vi "Chart_Generation_Formula.vi"(3 "Max Voltage":dbl, 7 "error in (no error)":errorcluster, 8 "Start":bool, 9 "CGF_Input":refnum<vi>, 10 "Polarity for Max Voltage":u16(ring) items=["Positive", "Negative"], 11 "Type of Chart":u16(ring) items=[" Crude Semi-Log (Short)", "Crude Semi-Log (Long)", "Bi-directional Crude Semi-Log (Short)", "Bi-directional Crude Semi-Log (Long)"]) -> (0 "Result - Test Voltages Array":dbl[](array[numeric]), 1 "~~ FINISH ~~":bool, 5 "error out":errorcluster)   [LabVIEW 2020]
uses:
  Global 1.vi
panel:
  out "Array Size":i32
  out "BiD : Test Voltages <OUTPUT>":dbl[](array[numeric])
  out "first subarray : PosTestV":dbl[](array[numeric])
  out "reversed array : NegTestV":dbl[](array[numeric])
  out "Flag Formula LCLC":bool
  out "Flag Formula SCLC":bool
  out "Checking NumberOfVoltages":i32
  out "DONE SUB Bi-LCLC":bool
  in  "SUB Bi-LCLC":bool
  out "DONE SUB Bi-SCLC":bool
  in  "SUB Bi-SCLC":bool
  out "BIDIRECTIONAL = FINISH Formulating Test Voltages":bool
  out "Bi-directional Crude Semi-Log (Long)":bool
  out "Bi-directional Crude Semi-Log (Short)":bool
  out "Crude Semi-Log (Long)":bool
  out "Crude Semi-Log (Short)":bool
  out "NegativeVoltages[256]":dbl[](array[numeric])
  out "Negative value":dbl
  in  "NumberOfVoltages":i32
  out "DONE SUB LCLC":bool
  in  "SUB LCLC":bool
  out "UNIDIRECTIONAL - FINISH Formulating Test Voltages":bool
  out "DONE SUB SCLC":bool
  in  "SUB SCLC":bool
  out "UniD : Test Voltages <OUTPUT>":dbl[](array[numeric])
  out "Checking Value of X":i32
  out "PositiveVoltages[256]":dbl[](array[numeric])
  in  "x":i32
  in  "VRmax":dbl
  # "Type of Chart :\n\n1) Linear -  < not applied here > < directly in Generation Report VI >\n2) Crude Semi-Log (Short) -----------------------> 0 \n3) Crude Semi-Log (Long) -----------------------> 1\n4) Bi-directional Crude Semi-Log (Short) --------> 2\n5) Bi-directional Crude Semi-Log (Long) --------> 3"
  # "FOR"
  # "Bi-directional Crude Semi-Log (Short)"
  # "Bi-directional Crude Semi-Log (Long)"
  # "Polarity is applied for \nmaximum voltage only,\nno mention of minimum\nin QuickBasic Code"
  # "Polarity : \n1 = \"negative\" ; 0 = \"positive\""
  # "Max Voltage is the actual\nmaximum voltage from\ndatasheet, therefore,\nmust put (-) if negative"
  # "VRmax is for calculation purpose"
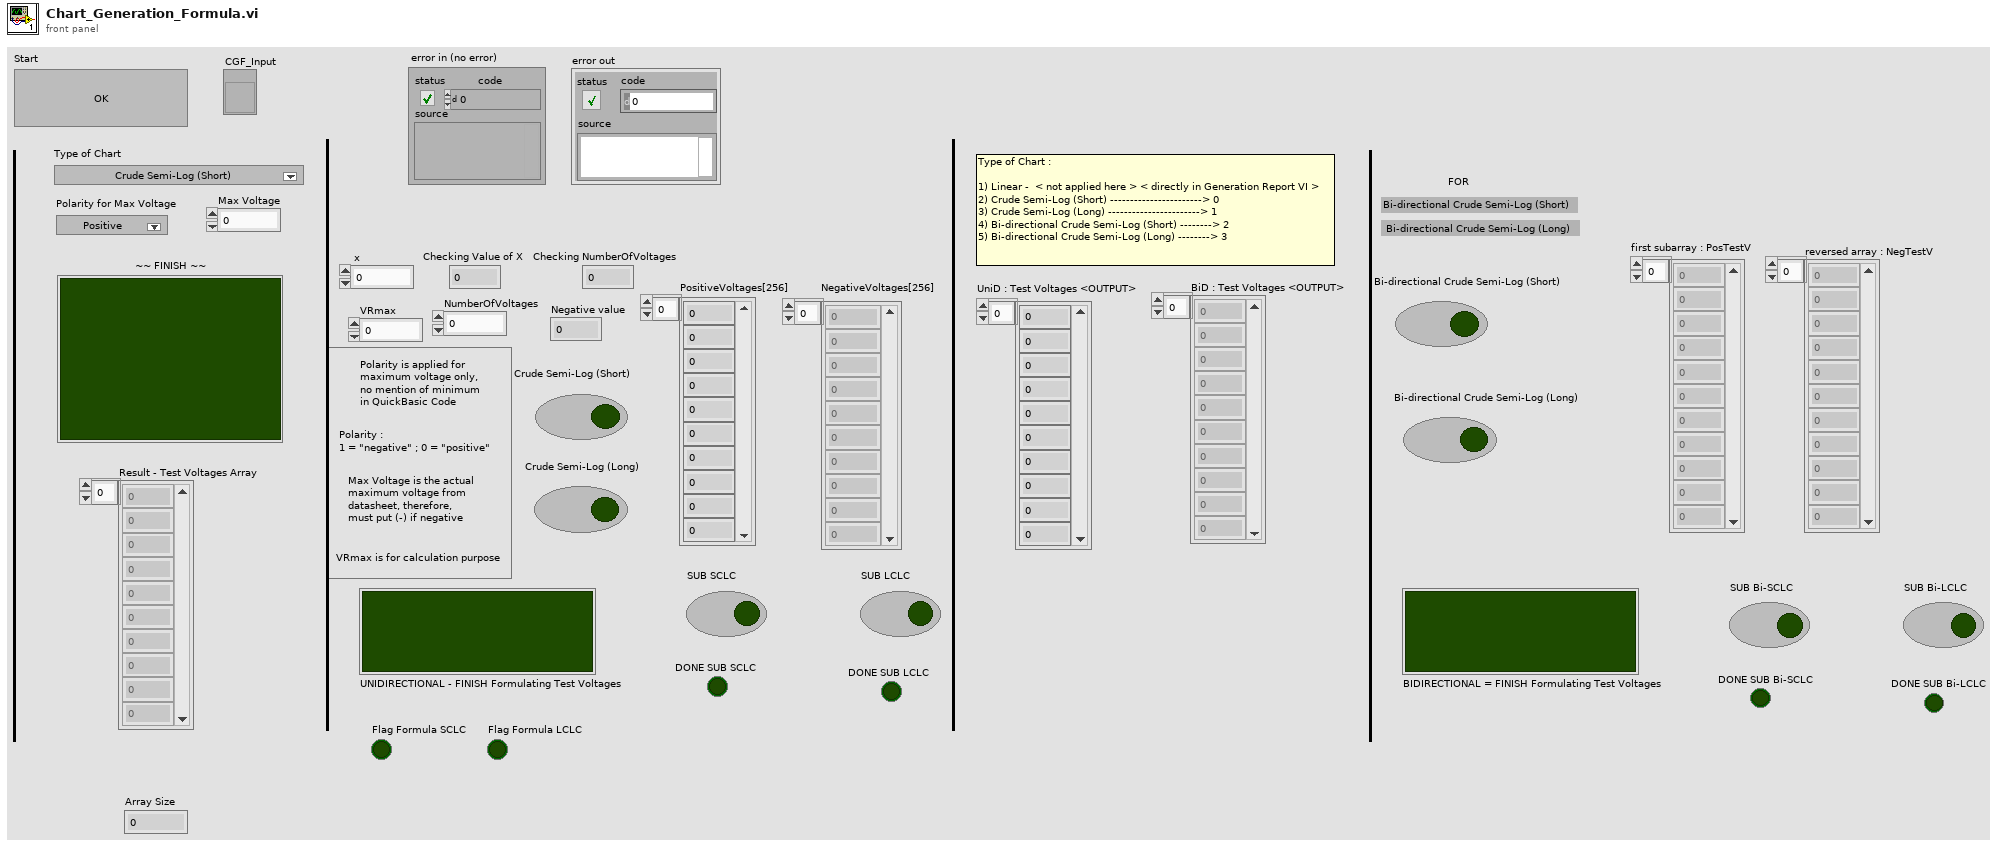
[diagram p1: front panel]
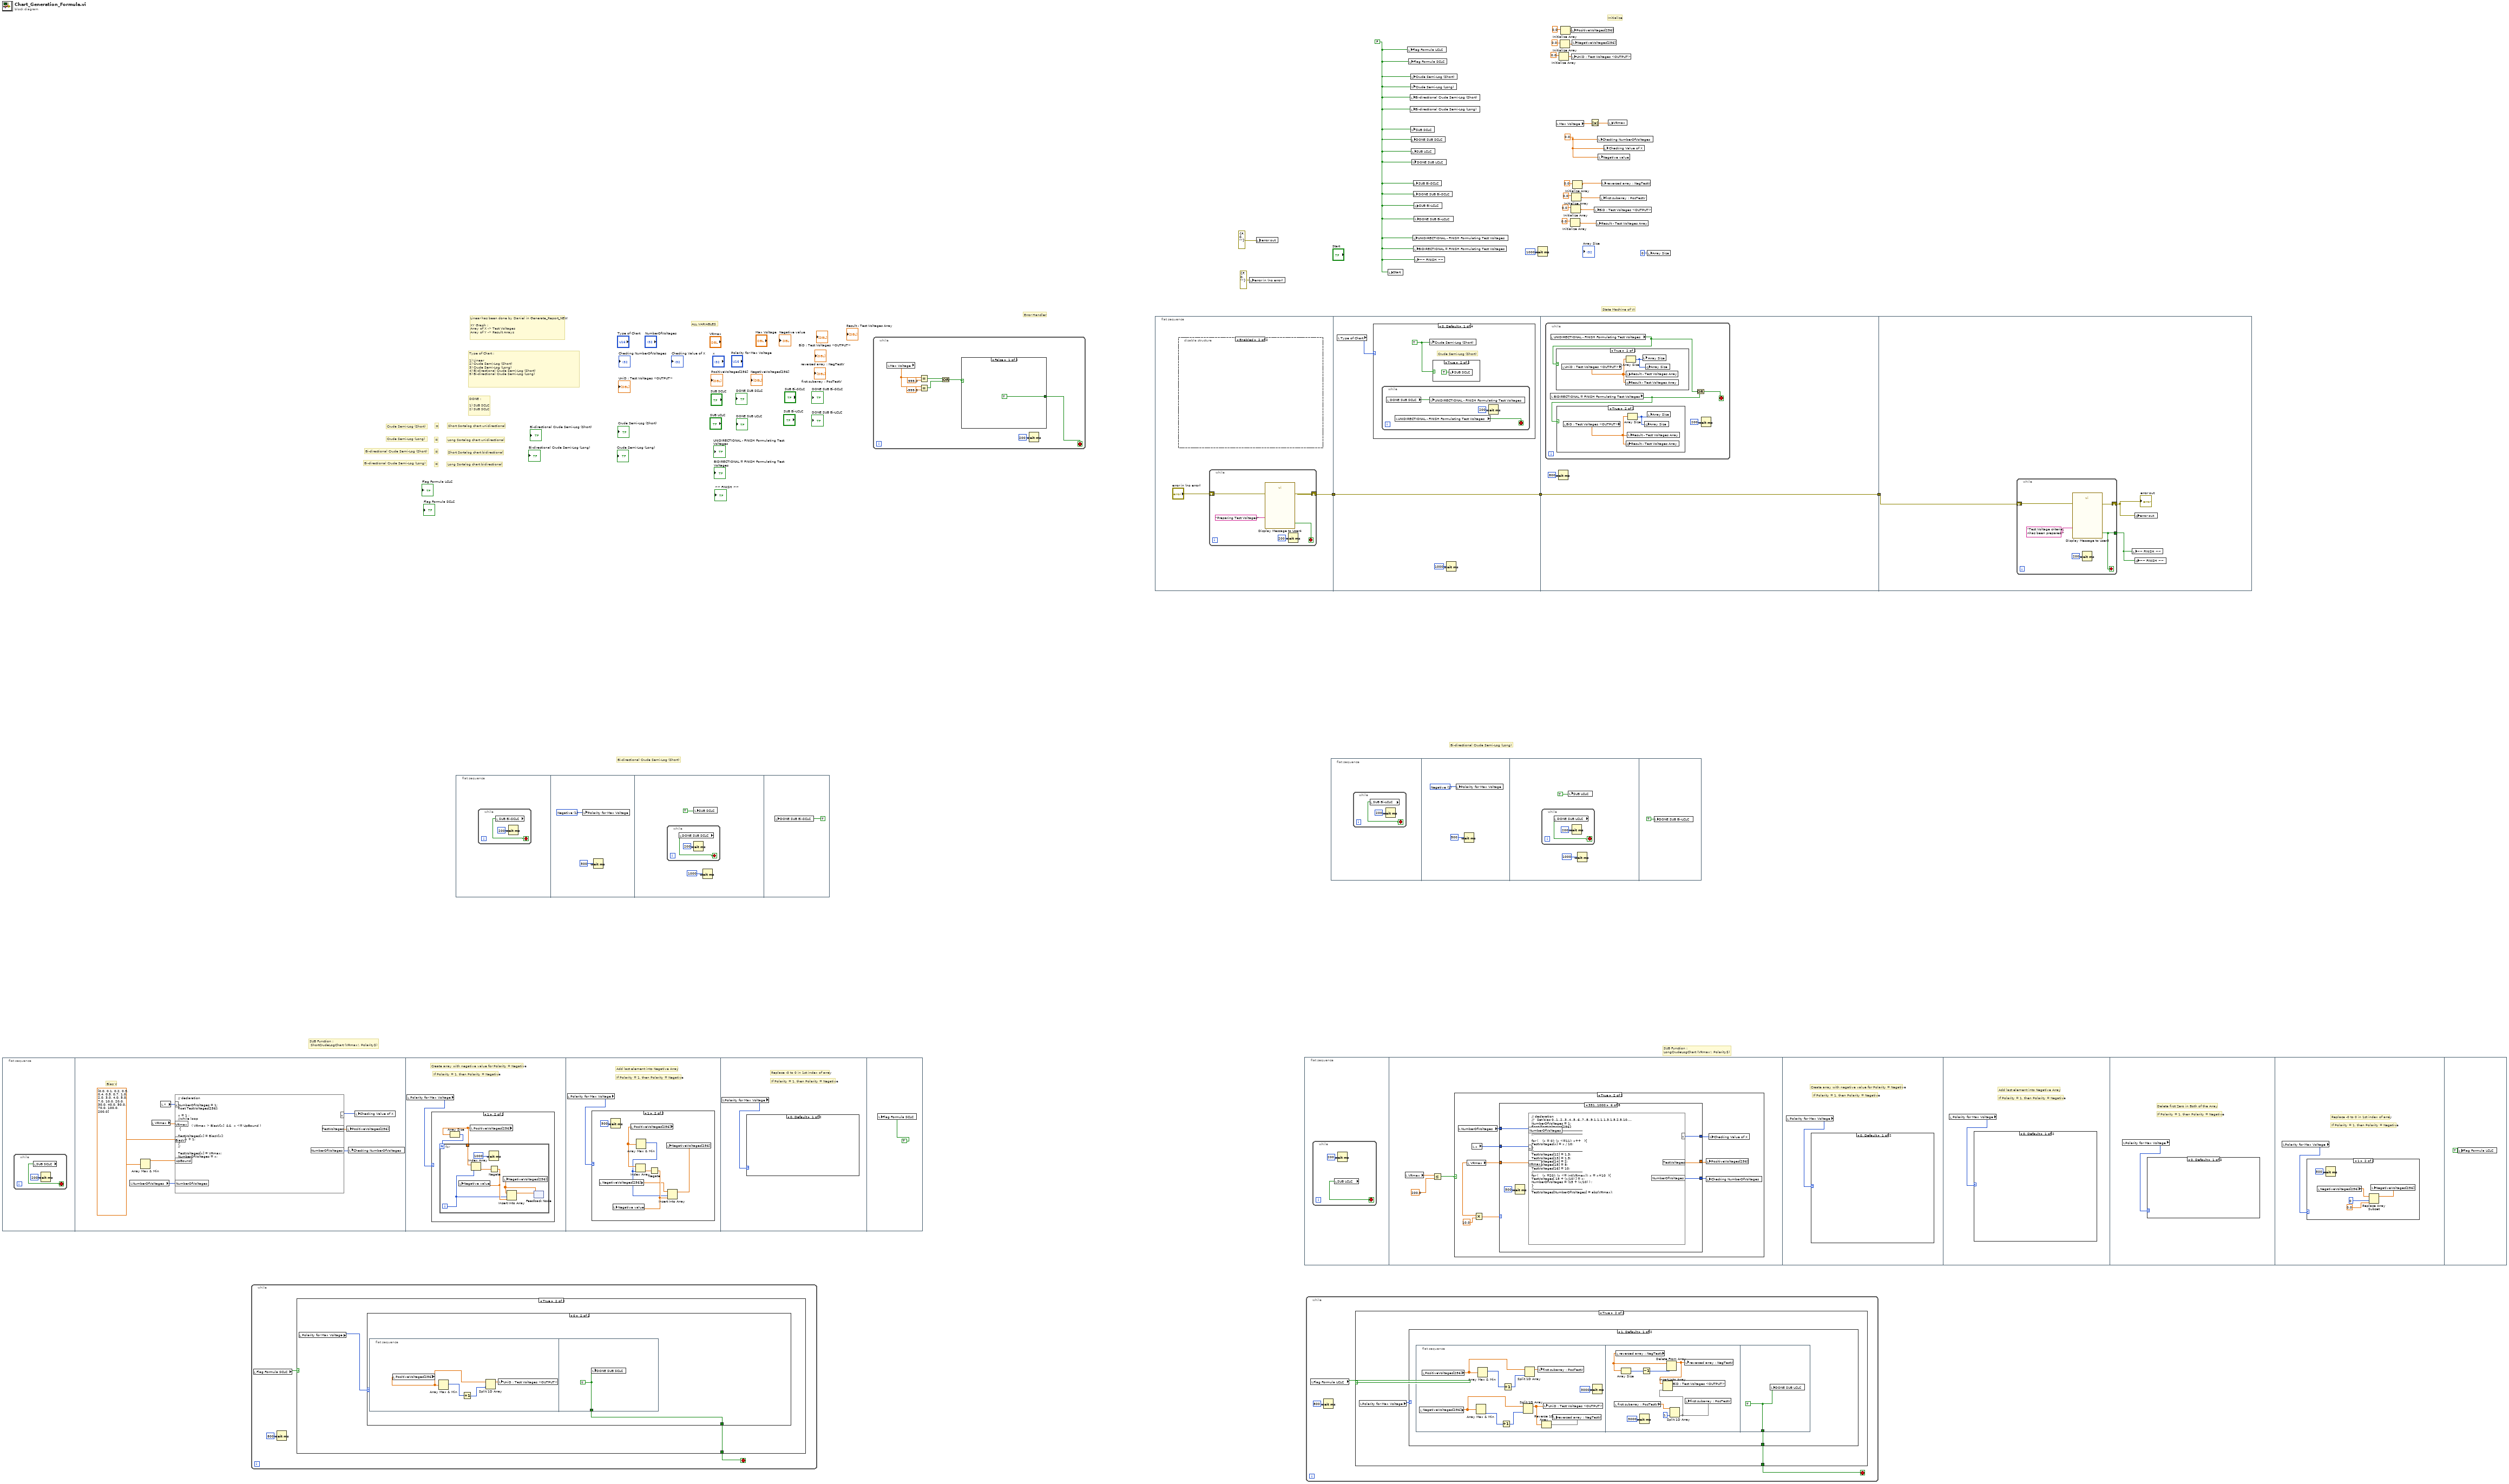
[diagram p0: block diagram]
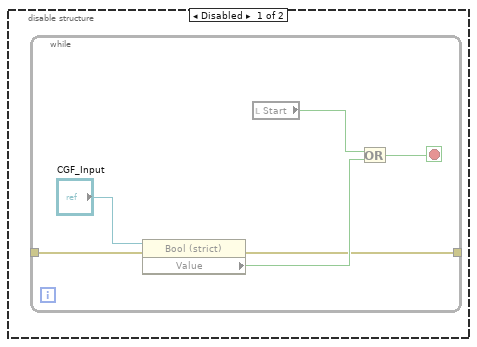
[diagram p2: hidden frame]
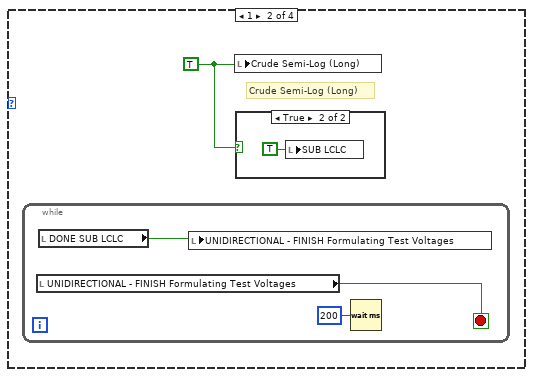
[diagram p4: hidden frame]
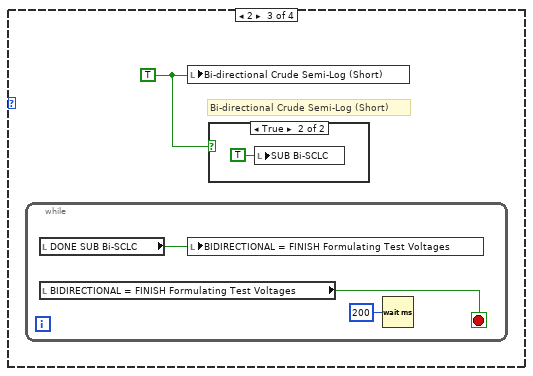
[diagram p6: hidden frame]
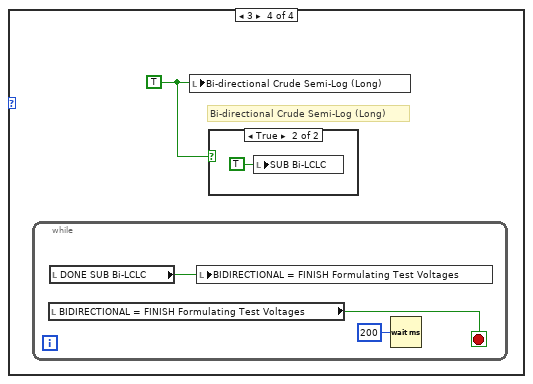
[diagram p8: hidden frame]
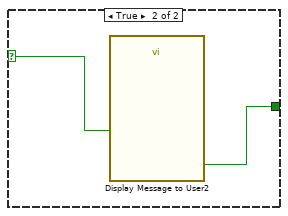
[diagram p12: hidden frame]
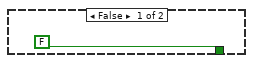
[diagram p13: hidden frame]
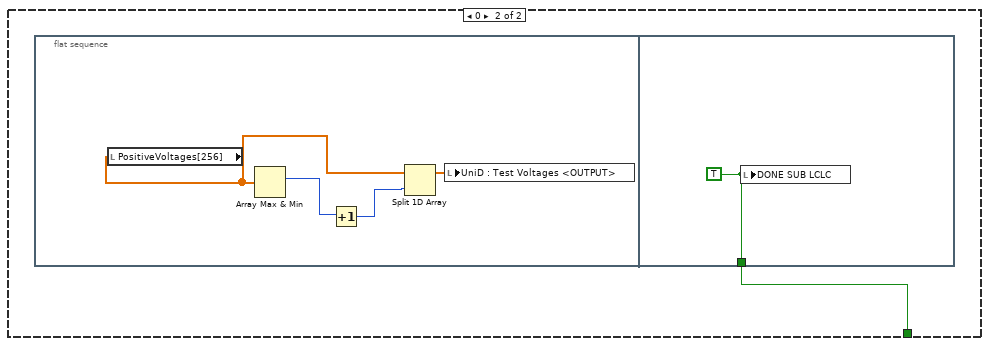
[diagram p14: hidden frame]
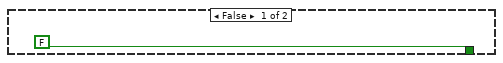
[diagram p15: hidden frame]
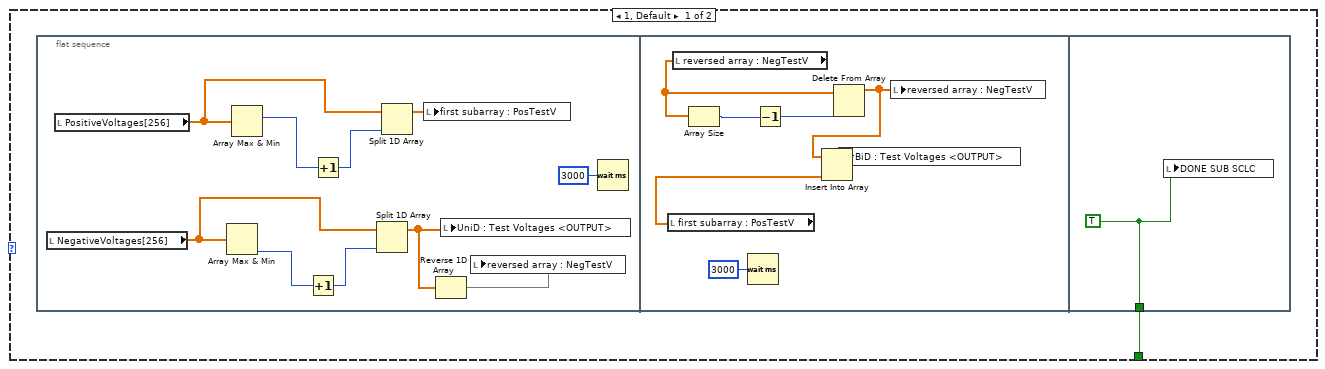
[diagram p16: hidden frame]
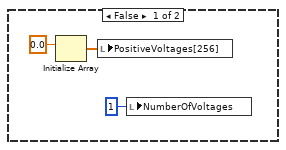
[diagram p17: hidden frame]
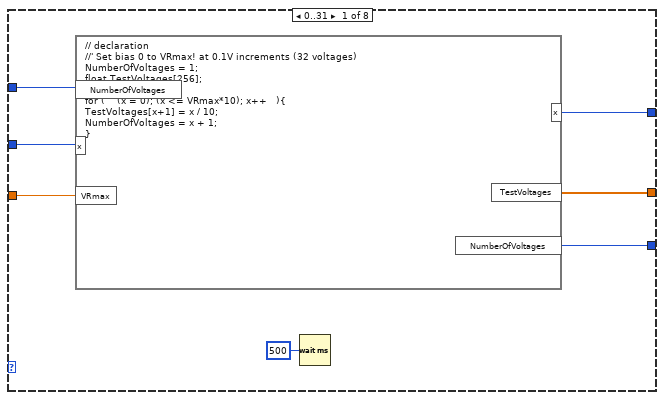
[diagram p18: hidden frame]
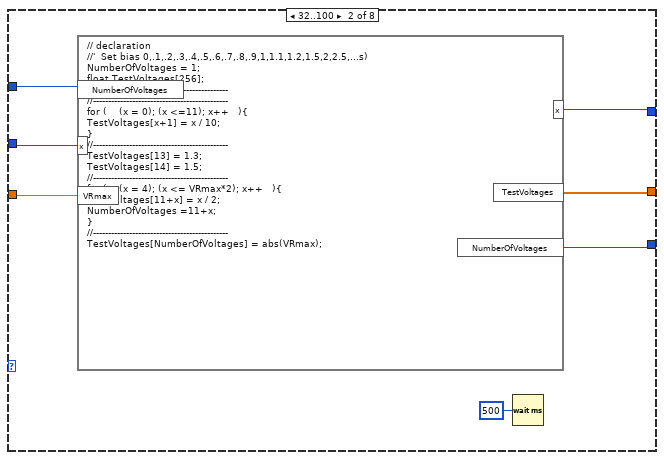
[diagram p19: hidden frame]
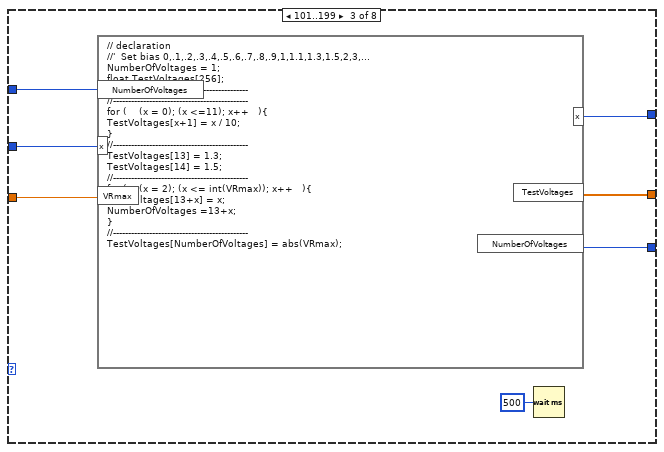
[diagram p20: hidden frame]
diagram:
  w16 = 0.0
  w3 = FALSE
  # "Bi-directional Crude Semi-Log (Long)"
  # "Bi-directional Crude Semi-Log (Short)"
  # "Initialize"
  # "State Machine of VI"
  # "Error Handler"
  # "Long Sortalog chart bidirectional"
  # "="
  # "Short Sortalog chart bidirectional"
  # "="
  # "="
  # "="
  # "Long Sortalog chart unidirectional"
  # "Short Sortalog chart unidirectional"
  # "Bi-directional Crude Semi-Log (Long)"
  # "Bi-directional Crude Semi-Log (Short)"
  # "Crude Semi-Log (Long)"
  # "Crude Semi-Log (Short)"
  # "DONE :\n\n1) SUB SCLC\n2) SUB SCLC"
  # "ALL VARIABLES"
  # "SUB Function :\nLongCrudeLogChart (VRmax!, Polarity$)"
  # "SUB Function :\n ShortCrudeLogChart (VRmax!, Polarity$)"
  # "Type of Chart :\n\n1) Linear\n2) Crude Semi-Log (Short) \n3) Crude Semi-Log (Long)\n4) Bi-directional Crude Semi-Log (Short)\n5) Bi-directional Crude Semi-Log (Long)"
  # "Linear has been done by Daniel in Generate_Report_NEW\n\nXY Graph : \nArray of X -> Test Voltages\nArray of Y -> Result Arrays"
  n1 = flat-sequence {
    frame #0 {
      n2 = while {
        stop <- w27 stop-if-true
        n3 = local read "SUB SCLC"() -> (w27:bool)
        n4 = Wait (ms)(milliseconds to wait=u32 200) -> ()  [unwired: 1 out]
      }
    }
    frame #1 {
      w35 = dbl[] [0.0, 0.1, 0.2, 0.3, 0.4, 0.5, 0.7, 1.0, 2.0, 3.0, 4.0, 5.0, 7.0, 10.0, 20.0, 30.0, 40.0, 50.0, 70.0, 100.0, 200.0]
      # "Bias V"
      n5 = local read "NumberOfVoltages"() -> (w29:i32)
      n6 = Array Max & Min(array=w35) -> (max value=w34:dbl)  [unwired: 3 out]
      n7 = local read "VRmax"() -> (w32:dbl)
      n8 = local read "x"() -> (w33:i32)
      n9 = formula code="// declaration\n\nNumberOfVoltages = 1;\nfloat TestVoltages[256];\n\nx = 1 ;\n//while loop\n\n while   ( VRmax > BiasV[x]  &&  x <= UpBound ) \n {\n\nTestVoltages[x] = BiasV[x];\nx = x + 1;\n}\n//\n\nTestVoltages[x] = VRmax;\nNumberOfVoltages = x;"("x"=w33, "VRmax"=w32, "BiasV"=w35, "NumberOfVoltages"=w29, "UpBound"=w34) -> ("x"=w31:i32, "TestVoltages"=w30:dbl[], "NumberOfVoltages"=w28:i32)
      n10 = local write "PositiveVoltages[256]"(w30) -> ()
      n11 = local write "Checking NumberOfVoltages"(w28) -> ()
      n12 = local write "Checking Value of X"(w31) -> ()
    }
    frame #2 {
      # "If Polarity = 1, then Polarity = Negative"
      # "Create array with negative value for Polarity = Negative"
      n13 = local read "Polarity for Max Voltage"() -> (w36:u16)
      n14 = case shown="1" w36 {
        frame 0, Default {
        }
        frame 1 {
          n15 = local read "PositiveVoltages[256]"() -> (w38:dbl[])
          n16 = Array Size(array=w38) -> (size(s)=w37:i32)
          n17 = for {
            N: w37 -> [_]
            tunnel: w38 -> [w44]
            i -> [w41]
            n18 = Index Array(array=w44, index=w41) -> (element=w45:dbl)
            n19 = Wait (ms)(milliseconds to wait=u32 1000) -> ()  [unwired: 1 out]
            n20 = Negate(x=w45) -> (-x=w42:dbl)
            n21 = local write "Negative value"(w42) -> ()
            n22 = feedback #1() -> (w40:dbl[])  [unwired: 1 in]
            n23 = local write "NegativeVoltages[256]"(w40) -> ()
            n24 = Insert Into Array(array=w40, index=w41, new element=w42) -> (w39:dbl[])
            n25 = feedback-in #1(w39) -> ()
          }
        }
      }
    }
    frame #3 {
      # "Add last element into Negative Array"
      # "If Polarity = 1, then Polarity = Negative"
      n26 = local read "Polarity for Max Voltage"() -> (w46:u16)
      n27 = case shown="1" w46 {
        frame 0, Default {
        }
        frame 1 {
          n28 = local read "NegativeVoltages[256]"() -> (w47:dbl[])
          n29 = Wait (ms)(milliseconds to wait=u32 500) -> ()  [unwired: 1 out]
          n30 = local read "PositiveVoltages[256]"() -> (w50:dbl[])
          n31 = Array Max & Min(array=w50) -> (max index (indices)=w49:i32)  [unwired: 3 out]
          n32 = Index Array(array=w50, index=w49) -> (element=w53:dbl)
          n33 = Negate(x=w53) -> (-x=w51:dbl)
          n34 = local write "Negative value"(w51) -> ()
          n35 = Insert Into Array(array=w47, index=w49, new element=w51) -> (w48:dbl[])
          n36 = local write "NegativeVoltages[256]"(w48) -> ()
        }
      }
    }
    frame #4 {
      # "Replace -0 to 0 in 1st index of array"
      # "If Polarity = 1, then Polarity = Negative"
      n37 = local read "Polarity for Max Voltage"() -> (w54:u16)
      n38 = case shown="0, Default" w54 {
        frame 0, Default {
        }
        frame 1 {
          n39 = local read "NegativeVoltages[256]"() -> (w58:dbl[])
          n40 = Wait (ms)(milliseconds to wait=u32 500) -> ()  [unwired: 1 out]
          n41 = Replace Array Subset(array=w58, new element=0.0 ("new element/subarray"), index=0) -> (w57:dbl[])
          n42 = local write "NegativeVoltages[256]"(w57) -> ()
        }
      }
    }
    frame #5 {
      n43 = local write "Flag Formula SCLC"(TRUE) -> ()
    }
  }
  n44 = while {
    stop <- w62 stop-if-true
    n45 = local read "Flag Formula SCLC"() -> (w63:bool)
    n46 = Wait (ms)(milliseconds to wait=u32 800) -> ()  [unwired: 1 out]
    n47 = case shown="True" w63 {
      tunnel: [FALSE ("FINISH CHART") w66] -> w62
      frame False {
      }
      frame True {
        n48 = local read "Polarity for Max Voltage"() -> (w65:u16)
        n49 = case shown="0" w65 {
          tunnel: [w67 w86] -> w66
          frame 1, Default {
            n50 = flat-sequence {
              tunnel: [w85] -> w67
              frame #0 {
                n51 = local read "NegativeVoltages[256]"() -> (w77:dbl[])
                n52 = local read "PositiveVoltages[256]"() -> (w71:dbl[])
                n53 = Array Max & Min(array=w77) -> (min index (indices)=w76:i32)  [unwired: 3 out]
                n54 = Array Max & Min(array=w71) -> (max index (indices)=w70:i32)  [unwired: 3 out]
                n55 = Increment(x=w76) -> (x+1=w73:i32)
                n56 = Increment(x=w70) -> (x+1=w72:i32)
                n57 = Split 1D Array(array=w77, index=w73) -> (first subarray=w74:dbl[])  [unwired: 1 out]
                n58 = Split 1D Array(array=w71, index=w72) -> (first subarray=w69:dbl[])  [unwired: 1 out]
                n59 = local write "first subarray : PosTestV"(w69) -> ()
                n60 = Reverse 1D Array(array=w74) -> (reversed array=w68:dbl[])
                n61 = local write "UniD : Test Voltages <OUTPUT>"(w74) -> ()
                n62 = local write "reversed array : NegTestV"(w68) -> ()
                n63 = Wait (ms)(milliseconds to wait=u32 3000) -> ()  [unwired: 1 out]
              }
              frame #1 {
                n64 = local read "first subarray : PosTestV"() -> (w84:dbl[])
                n65 = local read "reversed array : NegTestV"() -> (w82:dbl[])
                n66 = Array Size(array=w82) -> (size(s)=w81:i32)
                n67 = Wait (ms)(milliseconds to wait=u32 3000) -> ()  [unwired: 1 out]
                n68 = Decrement(x=w81) -> (x-1=w80:i32)
                n69 = Delete From Array(array=w82, index=w80) -> (array with subset deleted=w78:dbl[])  [unwired: 1 in, 1 out]
                n70 = Insert Into Array(array=w78, new element=w84) -> (w79:dbl[])  [unwired: 1 in]
                n71 = local write "BiD : Test Voltages <OUTPUT>"(w79) -> ()
                n72 = local write "reversed array : NegTestV"(w78) -> ()
              }
              frame #2 {
                w85 = TRUE ("FINISH CHART")
                n73 = local write "DONE SUB SCLC"(w85) -> ()
              }
            }
          }
          frame 0 {
            n74 = flat-sequence {
              tunnel: [w91] -> w86
              frame #0 {
                n75 = local read "PositiveVoltages[256]"() -> (w88:dbl[])
                n76 = Array Max & Min(array=w88) -> (max index (indices)=w90:i32)  [unwired: 3 out]
                n77 = Increment(x=w90) -> (x+1=w89:i32)
                n78 = Split 1D Array(array=w88, index=w89) -> (first subarray=w87:dbl[])  [unwired: 1 out]
                n79 = local write "UniD : Test Voltages <OUTPUT>"(w87) -> ()
              }
              frame #1 {
                w91 = TRUE ("FINISH CHART")
                n80 = local write "DONE SUB SCLC"(w91) -> ()
              }
            }
          }
        }
      }
    }
  }
  n81 = flat-sequence {
    frame #0 {
      n82 = while {
        stop <- w93 stop-if-true
        n83 = local read "SUB Bi-SCLC"() -> (w93:bool)
        n84 = Wait (ms)(milliseconds to wait=u32 200) -> ()  [unwired: 1 out]
      }
    }
    frame #1 {
      w95 = u16 1 items=["Positive", "Negative"] ("Polarity for Max Voltage")
      n85 = local write "Polarity for Max Voltage"(w95) -> ()
      n86 = Wait (ms)(milliseconds to wait=u32 500) -> ()  [unwired: 1 out]
    }
    frame #2 {
      n87 = while {
        stop <- w99 stop-if-true
        n88 = local read "DONE SUB SCLC"() -> (w99:bool)
        n89 = Wait (ms)(milliseconds to wait=u32 200) -> ()  [unwired: 1 out]
      }
      n90 = local write "SUB SCLC"(TRUE ("SUB SCLC")) -> ()
      n91 = Wait (ms)(milliseconds to wait=u32 1000) -> ()  [unwired: 1 out]
    }
    frame #3 {
      n92 = local write "DONE SUB Bi-SCLC"(TRUE ("DONE SUB Bi-SCLC")) -> ()
    }
  }
  n93 = while {
    stop <- w102 stop-if-true
    n94 = local read "Max Voltage"() -> (w104:dbl)
    n95 = Equal?(x=w104, y=999.0) -> (x = y?=w107:bool)
    n96 = Equal?(x=w104, y=-999.0) -> (x = y?=w106:bool)
    n97 = Or(x=w107, y=w106) -> (x .or. y?=w103:bool)
    n98 = case shown="False" w103 {
      selector: w103 -> [_ w111]
      tunnel: [TRUE w110] -> w102
      frame False {
      }
      frame True {
        n99 = call "Display Message to User2"("Enable"=w111) -> ("OK"=w110:bool)  [unwired: 9 in, 1 out]
      }
    }
    n100 = Wait (ms)(milliseconds to wait=u32 200) -> ()  [unwired: 1 out]
  }
  n101 = flat-sequence {
    tunnel: [w113] -> w1
    tunnel: [w125] -> w7
    tunnel: w1 -> [w125]
    tunnel: w7 -> [w148]
    tunnel: [w148] -> w2
    tunnel: w2 -> [w160]
    frame #0 {
      n102 = disable-structure shown="Enabled" {
        frame Disabled {
          n103 = while {
            tunnel: _ -> [w120]
            tunnel: [w119] -> _
            stop <- w123 stop-if-true
            n104 = property class="Bool (strict)"(reference="CGF_Input", error in=w120) -> (error out=w119:errorcluster, "Value"=w122:bool)  [unwired: 1 out]
            n105 = local read "Start"() -> (w124:bool)
            n106 = Or(x=w124, y=w122) -> (x .or. y?=w123:bool)
          }
        }
        frame Enabled {
        }
      }
      n107 = while {
        shift-right: [w116] -> w113
        shift-left: "error in (no error)" -> [w117]
        stop <- w114 stop-if-true
        n108 = call "Display Message to User4"("error in (no error)"=w117, "Message"="Preparing Test Voltages") -> ("error out"=w116:errorcluster, "OK"=w114:bool)  [unwired: 8 in]
        n109 = Wait (ms)(milliseconds to wait=u32 200) -> ()  [unwired: 1 out]
      }
    }
    frame #1 {
      n110 = local read "Type of Chart"() -> (w127:u16)
      n111 = case shown="0, Default" w127 {
        frame 0, Default {
          w128 = TRUE ("Crude Semi-Log (Short)")
          # "Crude Semi-Log (Short)"
          n112 = while {
            stop <- w130 stop-if-true
            n113 = local read "DONE SUB SCLC"() -> (w131:bool)
            n114 = local read "UNIDIRECTIONAL - FINISH Formulating Test Voltages"() -> (w130:bool)
            n115 = local write "UNIDIRECTIONAL - FINISH Formulating Test Voltages"(w131) -> ()
            n116 = Wait (ms)(milliseconds to wait=u32 200) -> ()  [unwired: 1 out]
          }
          n117 = local write "Crude Semi-Log (Short)"(w128) -> ()
          n118 = case shown="True" w128 {
            frame False {
            }
            frame True {
              n119 = local write "SUB SCLC"(TRUE ("SUB SCLC")) -> ()
            }
          }
        }
        frame 1 {
          w133 = TRUE ("Crude Semi-Log (Long)")
          # "Crude Semi-Log (Long)"
          n120 = while {
            stop <- w135 stop-if-true
            n121 = local read "UNIDIRECTIONAL - FINISH Formulating Test Voltages"() -> (w135:bool)
            n122 = local read "DONE SUB LCLC"() -> (w136:bool)
            n123 = local write "UNIDIRECTIONAL - FINISH Formulating Test Voltages"(w136) -> ()
            n124 = Wait (ms)(milliseconds to wait=u32 200) -> ()  [unwired: 1 out]
          }
          n125 = local write "Crude Semi-Log (Long)"(w133) -> ()
          n126 = case shown="True" w133 {
            frame False {
            }
            frame True {
              n127 = local write "SUB LCLC"(TRUE ("SUB SCLC")) -> ()
            }
          }
        }
        frame 2 {
          w138 = TRUE ("Bi-directional Crude Semi-Log (Short)")
          # "Bi-directional Crude Semi-Log (Short)"
          n128 = while {
            stop <- w140 stop-if-true
            n129 = local read "DONE SUB Bi-SCLC"() -> (w141:bool)
            n130 = local read "BIDIRECTIONAL = FINISH Formulating Test Voltages"() -> (w140:bool)
            n131 = local write "BIDIRECTIONAL = FINISH Formulating Test Voltages"(w141) -> ()
            n132 = Wait (ms)(milliseconds to wait=u32 200) -> ()  [unwired: 1 out]
          }
          n133 = local write "Bi-directional Crude Semi-Log (Short)"(w138) -> ()
          n134 = case shown="True" w138 {
            frame False {
            }
            frame True {
              n135 = local write "SUB Bi-SCLC"(TRUE ("SUB Bi-SCLC")) -> ()
            }
          }
        }
        frame 3 {
          w143 = TRUE ("Bi-directional Crude Semi-Log (Long)")
          # "Bi-directional Crude Semi-Log (Long)"
          n136 = while {
            stop <- w145 stop-if-true
            n137 = local read "BIDIRECTIONAL = FINISH Formulating Test Voltages"() -> (w145:bool)
            n138 = local read "DONE SUB Bi-LCLC"() -> (w146:bool)
            n139 = local write "BIDIRECTIONAL = FINISH Formulating Test Voltages"(w146) -> ()
            n140 = Wait (ms)(milliseconds to wait=u32 200) -> ()  [unwired: 1 out]
          }
          n141 = local write "Bi-directional Crude Semi-Log (Long)"(w143) -> ()
          n142 = case shown="True" w143 {
            frame False {
            }
            frame True {
              n143 = local write "SUB Bi-LCLC"(TRUE ("SUB Bi-LCLC")) -> ()
            }
          }
        }
      }
      n144 = Wait (ms)(milliseconds to wait=u32 1000) -> ()  [unwired: 1 out]
    }
    frame #2 {
      n145 = while {
        stop <- w153 stop-if-true
        n146 = local read "BIDIRECTIONAL = FINISH Formulating Test Voltages"() -> (w151:bool)
        n147 = local read "UNIDIRECTIONAL - FINISH Formulating Test Voltages"() -> (w152:bool)
        n148 = case shown="True" w152 {
          frame False {
          }
          frame True {
            n149 = local read "UniD : Test Voltages <OUTPUT>"() -> (w157:dbl[])
            n150 = global write "Global 1.vi" "Result - Test Voltages Array"(w157) -> ()
            n151 = Array Size(array=w157) -> (size(s)=w156:i32)
            n152 = local write "Result - Test Voltages Array"(w157) -> ()
            n153 = local write "Array Size"(w156) -> ()
            n154 = global write "Global 1.vi" "Array Size"(w156) -> ()
          }
        }
        n155 = case shown="True" w151 {
          frame False {
          }
          frame True {
            n156 = local read "BiD : Test Voltages <OUTPUT>"() -> (w155:dbl[])
            n157 = global write "Global 1.vi" "Result - Test Voltages Array"(w155) -> ()
            n158 = local write "Result - Test Voltages Array"(w155) -> ()
            n159 = Array Size(array=w155) -> (size(s)=w154:i32)
            n160 = global write "Global 1.vi" "Array Size"(w154) -> ()
            n161 = local write "Array Size"(w154) -> ()
          }
        }
        n162 = Or(x=w152, y=w151) -> (x .or. y?=w153:bool)
        n163 = Wait (ms)(milliseconds to wait=u32 200) -> ()  [unwired: 1 out]
      }
      n164 = Wait (ms)(milliseconds to wait=u32 800) -> ()  [unwired: 1 out]
    }
    frame #3 {
      n165 = while {
        tunnel: [w161] -> w159
        shift-right: [w163] -> w158
        shift-left: w160 -> [w164]
        stop <- w161 stop-if-true
        n166 = call "Display Message to User3"("error in (no error)"=w164, "Message"="Test Voltage criteria\nhas been prepared.") -> ("error out"=w163:errorcluster, "OK"=w161:bool)  [unwired: 8 in]
        n167 = Wait (ms)(milliseconds to wait=u32 200) -> ()  [unwired: 1 out]
      }
      "error out" <- w158
      n168 = local write "~~ FINISH ~~"(w159) -> ()
      n169 = global write "Global 1.vi" "error out"(w158) -> ()
      n170 = global write "Global 1.vi" "~~ FINISH ~~"(w159) -> ()
    }
  }
  n171 = local write "error in (no error)"(errorcluster {"status"=FALSE, "code"=0, "source"=""} ("error in (no error)")) -> ()
  n172 = local write "error out"(errorcluster {"status"=FALSE, "code"=0, "source"=""} ("error out")) -> ()
  n173 = flat-sequence {
    frame #0 {
      n174 = while {
        stop <- w167 stop-if-true
        n175 = local read "SUB LCLC"() -> (w167:bool)
        n176 = Wait (ms)(milliseconds to wait=u32 200) -> ()  [unwired: 1 out]
      }
    }
    frame #1 {
      n177 = local read "VRmax"() -> (w169:dbl)
      n178 = Less Or Equal?(x=w169, y=200.0) -> (x <= y?=w170:bool)
      n179 = case shown="True" w170 {
        frame False {
          n180 = Initialize Array(0.0 ("element")) -> (w172:dbl[])  [unwired: 1 in]
          n181 = local write "PositiveVoltages[256]"(w172) -> ()
          n182 = local write "NumberOfVoltages"(1 ("NumberOfVoltages")) -> ()
        }
        frame True {
          n183 = local read "NumberOfVoltages"() -> (w176:i32)
          n184 = local read "VRmax"() -> (w179:dbl)
          n185 = local read "x"() -> (w177:i32)
          n186 = Multiply(x=w179, y=10.0) -> (x*y=w181:dbl)
          n187 = case shown="351..1000" w181 {
            tunnel: w179 -> [w188 w192 w200 w207 w214 w221 w228 _]
            tunnel: [w187 w194 w199 w206 w213 w220 w227 _] -> w178
            tunnel: w177 -> [w186 w193 w201 w208 w215 w222 w229 _]
            tunnel: w176 -> [w185 w195 w202 w209 w216 w223 w230 _]
            tunnel: [w183 w190 w197 w204 w211 w218 w225 _] -> w175
            tunnel: [w182 w189 w196 w203 w210 w217 w224 _] -> w174
            frame 0..31 {
              n188 = formula code="// declaration\n//' Set bias 0 to VRmax! at 0.1V increments (32 voltages)\nNumberOfVoltages = 1;\nfloat TestVoltages[256];\n\nfor (    (x = 0); (x <= VRmax*10); x++   ){\nTestVoltages[x+1] = x / 10;\nNumberOfVoltages = x + 1;\n}"("VRmax"=w188, "x"=w186, "NumberOfVoltages"=w185) -> ("TestVoltages"=w187:dbl[], "x"=w183:i32, "NumberOfVoltages"=w182:i32)
              n189 = Wait (ms)(milliseconds to wait=u32 500) -> ()  [unwired: 1 out]
            }
            frame 32..100 {
              n190 = formula code="// declaration\n//'  Set bias 0,.1,.2,.3,.4,.5,.6,.7,.8,.9,1,1.1,1.2,1.5,2,2.5,...s)\nNumberOfVoltages = 1;\nfloat TestVoltages[256];\n//---------------------------------------------\n//---------------------------------------------\nfor (    (x = 0); (x <=11); x++   ){\nTestVoltages[x+1] = x / 10;\n}\n//---------------------------------------------\nTestVoltages[13] = 1.3;\nTestVoltages[14] = 1.5;\n//---------------------------------------------\nfor (    (x = 4); (x <= VRmax*2); x++   ){\nTestVoltages[11+x] = x / 2;\nNumberOfVoltages =11+x;\n}\n//---------------------------------------------\nTestVoltages[NumberOfVoltages] = abs(VRmax);"("VRmax"=w192, "x"=w193, "NumberOfVoltages"=w195) -> ("TestVoltages"=w194:dbl[], "x"=w190:i32, "NumberOfVoltages"=w189:i32)
              n191 = Wait (ms)(milliseconds to wait=u32 500) -> ()  [unwired: 1 out]
            }
            frame 101..199 {
              n192 = formula code="// declaration\n//'  Set bias 0,.1,.2,.3,.4,.5,.6,.7,.8,.9,1,1.1,1.3,1.5,2,3,...\nNumberOfVoltages = 1;\nfloat TestVoltages[256];\n//---------------------------------------------\n//---------------------------------------------\nfor (    (x = 0); (x <=11); x++   ){\nTestVoltages[x+1] = x / 10;\n}\n//---------------------------------------------\nTestVoltages[13] = 1.3;\nTestVoltages[14] = 1.5;\n//---------------------------------------------\nfor (    (x = 2); (x <= int(VRmax)); x++   ){\nTestVoltages[13+x] = x;\nNumberOfVoltages =13+x;\n}\n//---------------------------------------------\nTestVoltages[NumberOfVoltages] = abs(VRmax);"("VRmax"=w200, "x"=w201, "NumberOfVoltages"=w202) -> ("TestVoltages"=w199:dbl[], "x"=w197:i32, "NumberOfVoltages"=w196:i32)
              n193 = Wait (ms)(milliseconds to wait=u32 500) -> ()  [unwired: 1 out]
            }
            frame 200..300 {
              n194 = formula code="// declaration\n//'  Set bias 0,.1,.2,.3,.4,.5,.6,.7,.8,.9,1,1.1,1.3,1.5,2,3,...\nNumberOfVoltages = 1;\nfloat TestVoltages[256];\n//---------------------------------------------\n//---------------------------------------------\nfor (    (x = 0); (x<=11); x++   ){\nTestVoltages[x+1] = x / 10;\n}\n//---------------------------------------------\nTestVoltages[13] = 1.3;\nTestVoltages[14] = 1.5;\n//---------------------------------------------\nfor (    (x = 2); (x <= int(VRmax)); x=x+2   ){\nTestVoltages[14+ x/2] = x;\nNumberOfVoltages =14+ x/2;\n}\n//---------------------------------------------\nTestVoltages[NumberOfVoltages] = abs(VRmax);"("VRmax"=w207, "x"=w208, "NumberOfVoltages"=w209) -> ("TestVoltages"=w206:dbl[], "x"=w204:i32, "NumberOfVoltages"=w203:i32)
              n195 = Wait (ms)(milliseconds to wait=u32 500) -> ()  [unwired: 1 out]
            }
            frame 301..350 {
              n196 = formula code="// declaration\n//'  Set bias 0,.1,.2,.3,.4,.5,.6,.7,.8,.9,1,1.1,1.3,1.5,2,5,10,...\nNumberOfVoltages = 1;\nfloat TestVoltages[256];\n//---------------------------------------------\n//---------------------------------------------\nfor (    (x = 0); (x <=11); x++   ){\nTestVoltages[x+1] = x / 10;\n}\n//---------------------------------------------\nTestVoltages[13] = 1.3;\nTestVoltages[14] = 1.5;\nTestVoltages[15] = 2;\n//---------------------------------------------\nfor (    (x =5); (x <= int(VRmax)); x=x+5   ){\nTestVoltages[15+ x/5] = x;\nNumberOfVoltages =15+ x/5;\n}\n//---------------------------------------------\nTestVoltages[NumberOfVoltages] = abs(VRmax);"("VRmax"=w214, "x"=w215, "NumberOfVoltages"=w216) -> ("TestVoltages"=w213:dbl[], "x"=w211:i32, "NumberOfVoltages"=w210:i32)
              n197 = Wait (ms)(milliseconds to wait=u32 500) -> ()  [unwired: 1 out]
            }
            frame 351..1000 {
              n198 = Wait (ms)(milliseconds to wait=u32 500) -> ()  [unwired: 1 out]
              n199 = formula code="// declaration\n//'  Set bias 0,.1,.2,.3,.4,.5,.6,.7,.8,.9,1,1.1,1.3,1.5,2,5,10,...\nNumberOfVoltages = 1;\nfloat TestVoltages[256];\n//---------------------------------------------\n//---------------------------------------------\n\nfor (    (x = 0); (x <=11); x++   ){\nTestVoltages[x] = x / 10;\n}\n//---------------------------------------------\nTestVoltages[12] = 1.3;\nTestVoltages[13] = 1.5;\nTestVoltages[14] = 2;\nTestVoltages[15] = 5;\nTestVoltages[16] = 10;\n//---------------------------------------------\nfor (    (x =20); (x <= int(VRmax)); x = x+10  ){\nTestVoltages[ 15 + (x/10) ] = x;\nNumberOfVoltages = (15 + (x/10) ) ;\n}\n//---------------------------------------------\nTestVoltages[NumberOfVoltages] = abs(VRmax);"("VRmax"=w221, "x"=w222, "NumberOfVoltages"=w223) -> ("TestVoltages"=w220:dbl[], "x"=w218:i32, "NumberOfVoltages"=w217:i32)
            }
            frame 1001..2000 {
              n200 = Wait (ms)(milliseconds to wait=u32 500) -> ()  [unwired: 1 out]
              n201 = formula code="// declaration\n//'  Set bias 0,.1,.2,.3,.4,.5,.6,.7,.8,.9,1,1.1,1.3,1.5,2,5,10,...\nNumberOfVoltages = 1;\nfloat TestVoltages[256];\n//---------------------------------------------\n//---------------------------------------------\nfor (    (x = 0); (x <=11); x++   ){\nTestVoltages[x+1] = x / 10;\n}\n//---------------------------------------------\nTestVoltages[13] = 1.3;\nTestVoltages[14] = 1.5;\nTestVoltages[15] = 2;\nTestVoltages[16] = 5;\nTestVoltages[17] = 10;\nTestVoltages[18] = 20;\n//---------------------------------------------\nfor (    (x =20); (x <= int(VRmax)); x=x+20  ){\nTestVoltages[17+ x/20] = x;\nNumberOfVoltages =17+ x/20;\n}\n//---------------------------------------------\nTestVoltages[NumberOfVoltages] = abs(VRmax);"("VRmax"=w228, "x"=w229, "NumberOfVoltages"=w230) -> ("TestVoltages"=w227:dbl[], "x"=w225:i32, "NumberOfVoltages"=w224:i32)
            }
            frame 2001.., Default {
              n202 = call "Display Message to User"() -> ()  [unwired: 10 in, 2 out]
            }
          }
          n203 = local write "PositiveVoltages[256]"(w178) -> ()
          n204 = local write "Checking NumberOfVoltages"(w174) -> ()
          n205 = local write "Checking Value of X"(w175) -> ()
        }
      }
    }
    frame #2 {
      # "If Polarity = 1, then Polarity = Negative"
      # "Create array with negative value for Polarity = Negative"
      n206 = local read "Polarity for Max Voltage"() -> (w231:u16)
      n207 = case shown="0, Default" w231 {
        frame 0, Default {
        }
        frame 1 {
          n208 = local read "PositiveVoltages[256]"() -> (w233:dbl[])
          n209 = Array Size(array=w233) -> (size(s)=w232:i32)
          n210 = for {
            N: w232 -> [_]
            tunnel: w233 -> [w239]
            i -> [w237]
            n211 = Index Array(array=w239, index=w237) -> (element=w240:dbl)
            n212 = Wait (ms)(milliseconds to wait=u32 1000) -> ()  [unwired: 1 out]
            n213 = Negate(x=w240) -> (-x=w234:dbl)
            n214 = local write "Negative value"(w234) -> ()
            n215 = feedback #2() -> (w235:dbl[])  [unwired: 1 in]
            n216 = local write "NegativeVoltages[256]"(w235) -> ()
            n217 = Insert Into Array(array=w235, index=w237, new element=w234) -> (w236:dbl[])
            n218 = feedback-in #2(w236) -> ()
          }
        }
      }
    }
    frame #3 {
      # "Add last element into Negative Array"
      # "If Polarity = 1, then Polarity = Negative"
      n219 = local read "Polarity for Max Voltage"() -> (w241:u16)
      n220 = case shown="0, Default" w241 {
        frame 0, Default {
        }
        frame 1 {
          n221 = local read "NegativeVoltages[256]"() -> (w242:dbl[])
          n222 = Wait (ms)(milliseconds to wait=u32 500) -> ()  [unwired: 1 out]
          n223 = local read "PositiveVoltages[256]"() -> (w245:dbl[])
          n224 = Array Max & Min(array=w245) -> (max index (indices)=w244:i32)  [unwired: 3 out]
          n225 = Index Array(array=w245, index=w244) -> (element=w248:dbl)
          n226 = Negate(x=w248) -> (-x=w246:dbl)
          n227 = local write "Negative value"(w246) -> ()
          n228 = Insert Into Array(array=w242, index=w244, new element=w246) -> (w243:dbl[])
          n229 = local write "NegativeVoltages[256]"(w243) -> ()
        }
      }
    }
    frame #4 {
      # "Delete first Zero in Both of the Array"
      # "If Polarity = 1, then Polarity = Negative"
      n230 = local read "Polarity for Max Voltage"() -> (w249:u16)
      n231 = case shown="0, Default" w249 {
        frame 0, Default {
        }
        frame 1 {
          n232 = local read "NegativeVoltages[256]"() -> (w252:dbl[])
          n233 = Wait (ms)(milliseconds to wait=u32 500) -> ()  [unwired: 1 out]
          n234 = Delete From Array(array=w252, index=0) -> (array with subset deleted=w251:dbl[])  [unwired: 1 in, 1 out]
          n235 = local write "NegativeVoltages[256]"(w251) -> ()
        }
      }
    }
    frame #5 {
      # "Replace -0 to 0 in 1st index of array"
      # "If Polarity = 1, then Polarity = Negative"
      n236 = local read "Polarity for Max Voltage"() -> (w254:u16)
      n237 = case shown="1" w254 {
        frame 0, Default {
        }
        frame 1 {
          n238 = local read "NegativeVoltages[256]"() -> (w258:dbl[])
          n239 = Wait (ms)(milliseconds to wait=u32 500) -> ()  [unwired: 1 out]
          n240 = Replace Array Subset(array=w258, new element=0.0 ("new element/subarray"), index=0) -> (w257:dbl[])
          n241 = local write "NegativeVoltages[256]"(w257) -> ()
        }
      }
    }
    frame #6 {
      n242 = local write "Flag Formula LCLC"(TRUE ("DONE SUB LCLC")) -> ()
    }
  }
  n243 = while {
    stop <- w262 stop-if-true
    n244 = local read "Flag Formula LCLC"() -> (w263:bool)
    n245 = Wait (ms)(milliseconds to wait=u32 800) -> ()  [unwired: 1 out]
    n246 = case shown="True" w263 {
      tunnel: [FALSE ("FINISH CHART") w266] -> w262
      frame False {
      }
      frame True {
        n247 = local read "Polarity for Max Voltage"() -> (w265:u16)
        n248 = case shown="1, Default" w265 {
          tunnel: [w267 w288] -> w266
          frame 1, Default {
            n249 = flat-sequence {
              tunnel: [w287] -> w267
              frame #0 {
                n250 = local read "NegativeVoltages[256]"() -> (w277:dbl[])
                n251 = local read "PositiveVoltages[256]"() -> (w271:dbl[])
                n252 = Array Max & Min(array=w277) -> (min index (indices)=w276:i32)  [unwired: 3 out]
                n253 = Array Max & Min(array=w271) -> (max index (indices)=w270:i32)  [unwired: 3 out]
                n254 = Increment(x=w276) -> (x+1=w273:i32)
                n255 = Increment(x=w270) -> (x+1=w272:i32)
                n256 = Split 1D Array(array=w277, index=w273) -> (first subarray=w274:dbl[])  [unwired: 1 out]
                n257 = Split 1D Array(array=w271, index=w272) -> (first subarray=w269:dbl[])  [unwired: 1 out]
                n258 = local write "first subarray : PosTestV"(w269) -> ()
                n259 = Reverse 1D Array(array=w274) -> (reversed array=w268:dbl[])
                n260 = local write "UniD : Test Voltages <OUTPUT>"(w274) -> ()
                n261 = local write "reversed array : NegTestV"(w268) -> ()
                n262 = Wait (ms)(milliseconds to wait=u32 3000) -> ()  [unwired: 1 out]
              }
              frame #1 {
                n263 = local read "first subarray : PosTestV"() -> (w280:dbl[])
                n264 = local read "reversed array : NegTestV"() -> (w285:dbl[])
                n265 = Array Size(array=w285) -> (size(s)=w284:i32)
                n266 = Wait (ms)(milliseconds to wait=u32 3000) -> ()  [unwired: 1 out]
                n267 = Decrement(x=w284) -> (x-1=w283:i32)
                n268 = Delete From Array(array=w285, index=w283) -> (array with subset deleted=w281:dbl[])  [unwired: 1 in, 1 out]
                n269 = Split 1D Array(array=w280, index=1) -> (second subarray=w278:dbl[])  [unwired: 1 out]
                n270 = Insert Into Array(array=w281, new element=w278) -> (w282:dbl[])  [unwired: 1 in]
                n271 = local write "BiD : Test Voltages <OUTPUT>"(w282) -> ()
                n272 = local write "reversed array : NegTestV"(w281) -> ()
                n273 = local write "first subarray : PosTestV"(w278) -> ()
              }
              frame #2 {
                w287 = TRUE ("FINISH CHART")
                n274 = local write "DONE SUB LCLC"(w287) -> ()
              }
            }
          }
          frame 0 {
            n275 = flat-sequence {
              tunnel: [w293] -> w288
              frame #0 {
                n276 = local read "PositiveVoltages[256]"() -> (w290:dbl[])
                n277 = Array Max & Min(array=w290) -> (max index (indices)=w292:i32)  [unwired: 3 out]
                n278 = Increment(x=w292) -> (x+1=w291:i32)
                n279 = Split 1D Array(array=w290, index=w291) -> (first subarray=w289:dbl[])  [unwired: 1 out]
                n280 = local write "UniD : Test Voltages <OUTPUT>"(w289) -> ()
              }
              frame #1 {
                w293 = TRUE ("FINISH CHART")
                n281 = local write "DONE SUB LCLC"(w293) -> ()
              }
            }
          }
        }
      }
    }
  }
  n282 = flat-sequence {
    frame #0 {
      n283 = while {
        stop <- w295 stop-if-true
        n284 = local read "SUB Bi-LCLC"() -> (w295:bool)
        n285 = Wait (ms)(milliseconds to wait=u32 200) -> ()  [unwired: 1 out]
      }
    }
    frame #1 {
      w297 = u16 1 items=["Positive", "Negative"] ("Polarity for Max Voltage")
      n286 = local write "Polarity for Max Voltage"(w297) -> ()
      n287 = Wait (ms)(milliseconds to wait=u32 500) -> ()  [unwired: 1 out]
    }
    frame #2 {
      n288 = while {
        stop <- w301 stop-if-true
        n289 = local read "DONE SUB LCLC"() -> (w301:bool)
        n290 = Wait (ms)(milliseconds to wait=u32 200) -> ()  [unwired: 1 out]
      }
      n291 = local write "SUB LCLC"(TRUE ("SUB SCLC")) -> ()
      n292 = Wait (ms)(milliseconds to wait=u32 1000) -> ()  [unwired: 1 out]
    }
    frame #3 {
      n293 = local write "DONE SUB Bi-LCLC"(TRUE ("DONE SUB Bi-SCLC")) -> ()
    }
  }
  n294 = local write "Start"(w3) -> ()
  n295 = local write "Flag Formula LCLC"(w3) -> ()
  n296 = local write "Flag Formula SCLC"(w3) -> ()
  n297 = local write "Bi-directional Crude Semi-Log (Short)"(w3) -> ()
  n298 = local write "Bi-directional Crude Semi-Log (Long)"(w3) -> ()
  n299 = local write "Crude Semi-Log (Short)"(w3) -> ()
  n300 = local write "Crude Semi-Log (Long)"(w3) -> ()
  n301 = local write "SUB SCLC"(w3) -> ()
  n302 = local write "DONE SUB SCLC"(w3) -> ()
  n303 = local write "SUB LCLC"(w3) -> ()
  n304 = local write "DONE SUB LCLC"(w3) -> ()
  n305 = local write "UNIDIRECTIONAL - FINISH Formulating Test Voltages"(w3) -> ()
  n306 = local write "SUB Bi-SCLC"(w3) -> ()
  n307 = local write "DONE SUB Bi-SCLC"(w3) -> ()
  n308 = local write "BIDIRECTIONAL = FINISH Formulating Test Voltages"(w3) -> ()
  n309 = local write "SUB Bi-LCLC"(w3) -> ()
  n310 = local write "DONE SUB Bi-LCLC"(w3) -> ()
  n311 = local write "~~ FINISH ~~"(w3) -> ()
  n312 = Wait (ms)(milliseconds to wait=u32 1000) -> ()  [unwired: 1 out]
  n313 = local read "Max Voltage"() -> (w23:dbl)
  n314 = Initialize Array(0.0 ("element")) -> (w20:dbl[])  [unwired: 1 in]
  n315 = Initialize Array(0.0 ("element")) -> (w21:dbl[])  [unwired: 1 in]
  n316 = Initialize Array(0.0 ("element")) -> (w19:dbl[])  [unwired: 1 in]
  n317 = Initialize Array(0.0 ("element")) -> (w10:dbl[])  [unwired: 1 in]
  n318 = Initialize Array(0.0 ("element")) -> (w11:dbl[])  [unwired: 1 in]
  n319 = local write "PositiveVoltages[256]"(w19) -> ()
  n320 = local write "UniD : Test Voltages <OUTPUT>"(w20) -> ()
  n321 = Initialize Array(0.0 ("element")) -> (w25:dbl[])  [unwired: 1 in]
  n322 = local write "NegativeVoltages[256]"(w21) -> ()
  n323 = Initialize Array(0.0 ("element")) -> (w24:dbl[])  [unwired: 1 in]
  n324 = Absolute Value(x=w23) -> (abs(x)=w22:dbl)
  n325 = local write "BiD : Test Voltages <OUTPUT>"(w11) -> ()
  n326 = local write "Result - Test Voltages Array"(w10) -> ()
  n327 = local write "Checking NumberOfVoltages"(w16) -> ()
  n328 = local write "Negative value"(w16) -> ()
  n329 = local write "first subarray : PosTestV"(w25) -> ()
  n330 = local write "reversed array : NegTestV"(w24) -> ()
  n331 = local write "Checking Value of X"(w16) -> ()
  n332 = local write "VRmax"(w22) -> ()
  n333 = local write "Array Size"(0 ("Array Size")) -> ()
